vi "Module Type.vi"(11 "SlowCalcs Module in":refnum<class "SlowCalcs Module.lvclass">) -> (2 "Module Type":string)   [LabVIEW 2020, in "VolatusCalcs.lvlib" / "SlowCalcs Module.lvclass"]
uses:
  SlowCalcs Module.lvclass
  SlowCalcs Module.lvclass/SlowCalcs Module.ctl
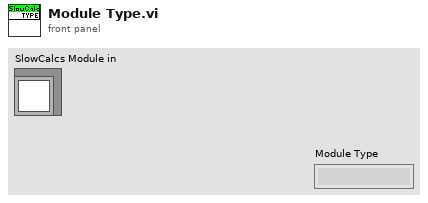
[diagram p1: front panel]
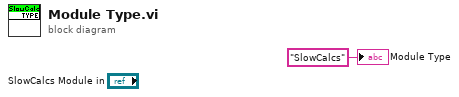
[diagram p0: block diagram]
diagram:
  "Module Type" <- "SlowCalcs" ("Module Type")
